vi "Decode DAQ Params.vi"(8 "error in (no error)":errorcluster, 11 "Data":variant) -> (0 "error out":errorcluster, 3 "Cluster":cluster{cluster{u16, string}, i32})   [LabVIEW 2026, in "TALOS.lvlib" / "Guardian.lvlib" / "Guardian.lvclass"]
uses:
  Guardian.lvclass
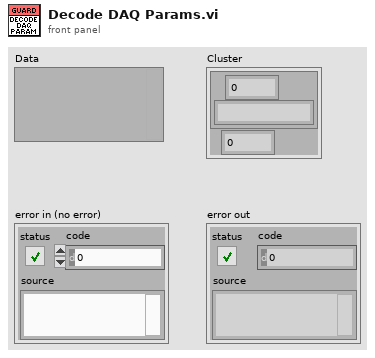
[diagram p1: front panel]
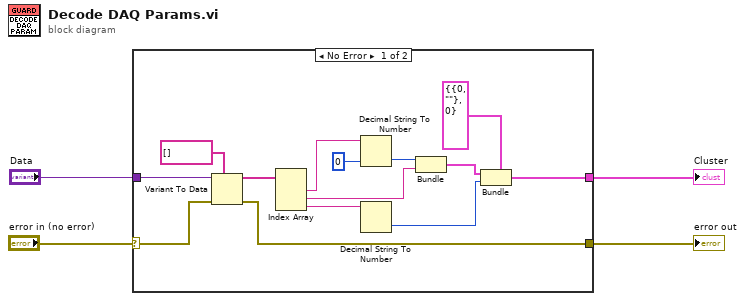
[diagram p0: block diagram]
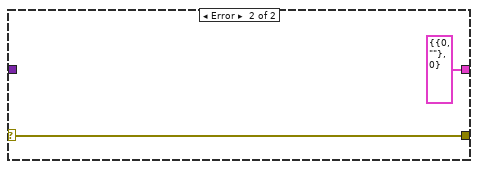
[diagram p2: hidden frame]
diagram:
  n1 = case shown="No Error" "error in (no error)" {
    selector: "error in (no error)" -> [w17 w20]
    tunnel: "Data" -> [w18 _]
    tunnel: [w6 w20] -> w2
    tunnel: [w7 cluster{cluster{u16, string}, i32} {{0, ""}, 0}] -> w1
    frame No Error {
      n2 = Variant To Data(error in=w17, type=string[] [], Variant=w18) -> (data=w5:string[], error out=w6:errorcluster)
      n3 = Index Array(array=w5) -> (element #1=w14:string, element #2=w9:string, element #3=w12:string)  [unwired: 3 in]
      n4 = Decimal String To Number(string=w14, default (0L)=u16 0 ("default (0 I32)")) -> (number=w13:u16)  [unwired: 1 in, 1 out]
      n5 = Decimal String To Number(string=w12) -> (number=w11:i32)  [unwired: 2 in, 1 out]
      n6 = Bundle(w13, "String"=w9) -> (w10:cluster{u16, "String":string})  [unwired: 1 in]
      n7 = Bundle(cluster=cluster{cluster{u16, string}, i32} {{0, ""}, 0}, w10, w11) -> (w7:cluster{cluster{u16, string}, i32})
    }
    frame Error {
    }
  }
  "error out" <- w2
  "Cluster" <- w1
